vi "Random_Color.vi"() -> (0 "Color":u32(colorbox))   [LabVIEW 2020]
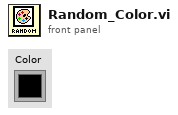
[diagram p1: front panel]
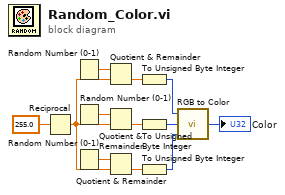
[diagram p0: block diagram]
diagram:
  n1 = Reciprocal(x=255.0) -> (1/x=w1:dbl)
  n2 = Random Number (0-1)() -> (number: 0 to 1=w3:dbl)
  n3 = Random Number (0-1)() -> (number: 0 to 1=w4:dbl)
  n4 = Random Number (0-1)() -> (number: 0 to 1=w5:dbl)
  n5 = Quotient & Remainder(x=w3, y=w1) -> (floor(x/y)=w7:dbl)  [unwired: 1 out]
  n6 = Quotient & Remainder(x=w4, y=w1) -> (floor(x/y)=w8:dbl)  [unwired: 1 out]
  n7 = Quotient & Remainder(x=w5, y=w1) -> (floor(x/y)=w9:dbl)  [unwired: 1 out]
  n8 = To Unsigned Byte Integer(number=w7) -> (unsigned 8bit integer=w10:u8)
  n9 = To Unsigned Byte Integer(number=w8) -> (unsigned 8bit integer=w11:u8)
  n10 = To Unsigned Byte Integer(number=w9) -> (unsigned 8bit integer=w12:u8)
  n11 = call <vilib>:"RGB to Color.vi"("B"=w12, "G"=w11, "R"=w10) -> ("Color"=→"Color":u32)
